vi "createSVEvent.vi"(7 "MonitorTaskTriggerEvent":refnum<class "HGF_Event.lvclass">, 8 "error in (no error)":errorcluster, 9 "Command(t)/\nSubscriber(f)":bool[](array[boolean]), 10 "TypeDescriptor":string[](array[string]), 11 "Array":refnum<k21>[](array[refnum])) -> (0 "error out":errorcluster, 2 "HGF Event":refnum<class "HGF_Event.lvclass">)   [LabVIEW 2012, in "HGF_SV.lvlib" / "HGF_SVEvent.lvclass"]
uses:
  HGF_SVEvent.lvclass
  HGF_BaseClasses/HGF_Event/HGF_Event.lvclass
  HGF_SVFactory/HGF_SVFactory.lvclass
  HGF_SVDataConverter/HGF_SVDataConverter.lvclass
  HGF_BaseClasses/HGF_PVSubscriber/HGF_PVSubscriber.lvclass
  HGF_BaseClasses/HGF_NetworkVisitor/HGF_NetworkVisitor.lvclass
  HGF_BaseClasses/HGF_PVBase/HGF_PVBase.lvclass
  HGF_BaseClasses/HGF_Factory/HGF_Factory.lvclass
  HGF_BaseClasses/HGF_NetworkEvent/HGF_NetworkEvent.lvclass/HGF_NetworkEvent.lvclass
  HGF_SVCommand/HGF_SVCommand.lvclass
  HGF_SVSubscriber/HGF_SVSubscriber.lvclass
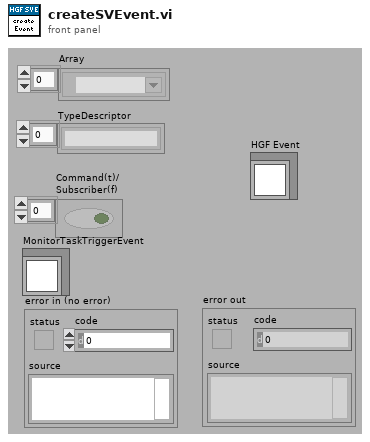
[diagram p1: front panel]
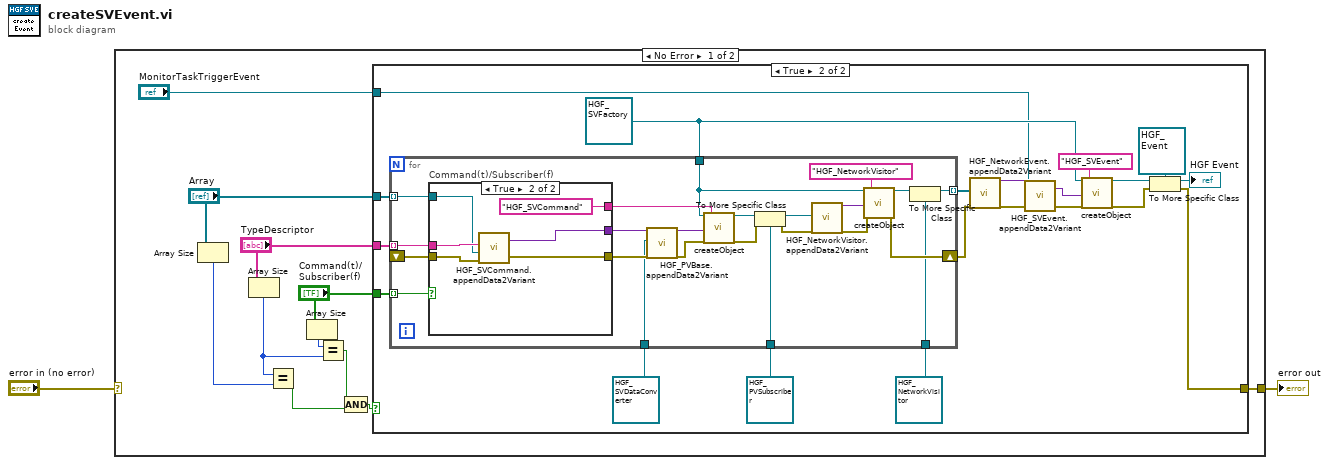
[diagram p0: block diagram]
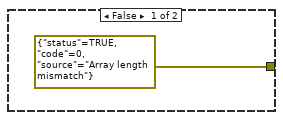
[diagram p2: hidden frame]
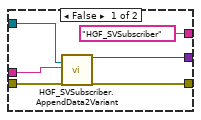
[diagram p3: hidden frame]
diagram:
  n1 = case shown="No Error" "error in (no error)" {
    selector: "error in (no error)" -> [_ w70]
    tunnel: [w5 w70] -> w2
    frame No Error {
      n2 = Array Size(array="Array") -> (size(s)=w9:i32)
      n3 = Array Size(array="TypeDescriptor") -> (size(s)=w10:i32)
      n4 = Equal?(x=w10, y=w9) -> (x = y?=w7:bool)
      n5 = Array Size(array="Command(t)/\nSubscriber(f)") -> (size(s)=w11:i32)
      n6 = Equal?(x=w11, y=w10) -> (x = y?=w8:bool)
      n7 = Compound Arithmetic op=AND(w8, w7) -> (w6:bool)
      n8 = case shown="True" w6 {
        tunnel: "Array" -> [_ w34]
        tunnel: "TypeDescriptor" -> [_ w33]
        tunnel: "Command(t)/\nSubscriber(f)" -> [_ w32]
        tunnel: "MonitorTaskTriggerEvent" -> [_ w15]
        tunnel: [errorcluster {"status"=TRUE, "code"=0, "source"="Array length mismatch"} ("error out") w17] -> w5
        frame False {
        }
        frame True {
          w22 = refnum<class "HGF_SVFactory.lvclass"> refnum ("DSC.lvlib:HGF_DSCFactory.lvclass")
          n9 = for {
            tunnel: w34 -> [w57] mode=indexing
            tunnel: w33 -> [w56] mode=indexing
            tunnel: w32 -> [w55] mode=indexing
            tunnel: w22 -> [w41]
            shift-right: [w39] -> w27
            shift-left: _ -> [w51]
            tunnel: refnum<class "HGF_SVDataConverter.lvclass"> refnum ("HGF_SV.lvlib:HGF_SVDataConverter.lvclass") -> [w47]
            tunnel: refnum<class "HGF_PVSubscriber.lvclass"> refnum ("HGF_BaseClasses.lvlib:HGF_PVSubscriber.lvclass") -> [w45]
            tunnel: [w35] -> w28 mode=indexing
            tunnel: refnum<class "HGF_NetworkVisitor.lvclass"> refnum ("HGF_BaseClasses.lvlib:HGF_NetworkVisitor.lvclass") -> [w36]
            n10 = case "Command(t)/Subscriber(f)" shown="True" w55 {
              tunnel: w57 -> [w58 w64]
              tunnel: w56 -> [w59 w69]
              tunnel: ["HGF_SVSubscriber" "HGF_SVCommand"] -> w54
              tunnel: [w62 w67] -> w49
              tunnel: w51 -> [w61 w66]
              tunnel: [w60 w65] -> w48
              frame False {
                n11 = call "HGF_SVSubscriber.AppendData2Variant.vi"("shared variable refnum"=w58, "typeDescriptor"=w59, "error in (no error)"=w61) -> ("dup initData"=w62:variant, "error out"=w60:errorcluster)  [unwired: 15 in]
              }
              frame True {
                n12 = call "HGF_SVCommand.appendData2Variant.vi"("error in (no error)"=w66, "shared variable refnum"=w64, "typeDescriptor"=w69) -> ("error out"=w65:errorcluster, "dup initData"=w67:variant)  [unwired: 1 in]
              }
            }
            n13 = call "HGF_PVBase.appendData2Variant.vi"("initData"=w49, "HGF_PVDataConverter"=w47, "error in (no error)"=w48) -> ("dup initData"=w50:variant, "error out"=w46:errorcluster)  [unwired: 15 out]
            n14 = call "createObject.vi"("HGF_Factory"=w41, "initializationData"=w50, "error in (no error)"=w46, "className"=w54) -> ("HGF_Object"=w52:refnum<class "HGF_Factory.lvclass">, "error out"=w53:errorcluster)  [unwired: 1 in, 13 out]
            n15 = To More Specific Class(target class=w45, reference=w52, error in=w53) -> (specific class reference=w44:refnum<class "HGF_PVSubscriber.lvclass">, error out=w43:errorcluster)
            n16 = call "HGF_NetworkVisitor.appendData2Variant.vi"("HGF_PVSubscriber"=w44, "error in (no error)"=w43) -> ("dup initData"=w42:variant, "error out"=w40:errorcluster)  [unwired: 1 in, 15 out]
            n17 = call "createObject.vi"("HGF_Factory"=w41, "initializationData"=w42, "error in (no error)"=w40, "className"="HGF_NetworkVisitor") -> ("HGF_Object"=w37:refnum<class "HGF_Factory.lvclass">, "error out"=w39:errorcluster)  [unwired: 1 in, 13 out]
            n18 = To More Specific Class(target class=w36, reference=w37) -> (specific class reference=w35:refnum<class "HGF_NetworkVisitor.lvclass">)  [unwired: 1 in, 1 out]
          }
          n19 = call "HGF_NetworkEvent.appendData2Variant.vi"("callbackVisitors"=w28, "error in (no error)"=w27) -> ("dup initData"=w25:variant, "error out"=w26:errorcluster)  [unwired: 1 in, 15 out]
          n20 = call "HGF_SVEvent.appendData2Variant.vi"("error in"=w26, "SV Monitor Trigger"=w15, "initData"=w25) -> ("error out"=w23:errorcluster, "dup initData"=w24:variant)
          n21 = call "createObject.vi"("HGF_Factory"=w22, "initializationData"=w24, "error in (no error)"=w23, "className"="HGF_SVEvent") -> ("HGF_Object"=w20:refnum<class "HGF_Factory.lvclass">, "error out"=w19:errorcluster)  [unwired: 1 in, 13 out]
          n22 = To More Specific Class(target class=refnum<class "HGF_Event.lvclass"> refnum ("HGF_BaseClasses.lvlib:HGF_Event.lvclass"), reference=w20, error in=w19) -> (specific class reference=→"HGF Event":refnum<class "HGF_Event.lvclass">, error out=w17:errorcluster)
        }
      }
    }
    frame Error {
    }
  }
  "error out" <- w2
